vi "ReadData_5782.vi"(10 "Buffer mode":T1, 11 "scope params":T2) -> (0 "error out":errorcluster, 1 "Num elements":i32, 2 "data":dbl[][](array[numeric]) format="%.2f", 3 "scope params out":T2)   [LabVIEW 2013]
uses:
  controls/scope_params_5782.ctl
  Utilities/Ticker/Ticker.lvclass
  Scope/controls/ScopeMode.ctl
  Config/FPGAref_5782.ctl
  FPGA/DataMode.ctl
  controls/5782_trigger_type.ctl
  Scope/controls/Data_display_mode.ctl
  <vilib>/rvi/interface/common/niFpgaWaitOnOcc.vi
  <vilib>/Utility/error.llb/Error Cluster From Error Code.vi
  <vilib>/rvi/errors/niLvFpgaAdjustHostInterfaceError.vi
  <vilib>/rvi/interface/nirviMethod/nirviMethod.xnode
  <vilib>/FPGAPlugInAG/Dynamic/niLvFpga_ReadFifo_Dynamic.vi
  <vilib>/rvi/errors/niLvFpgaMergeErrorWithErrorCode.vi
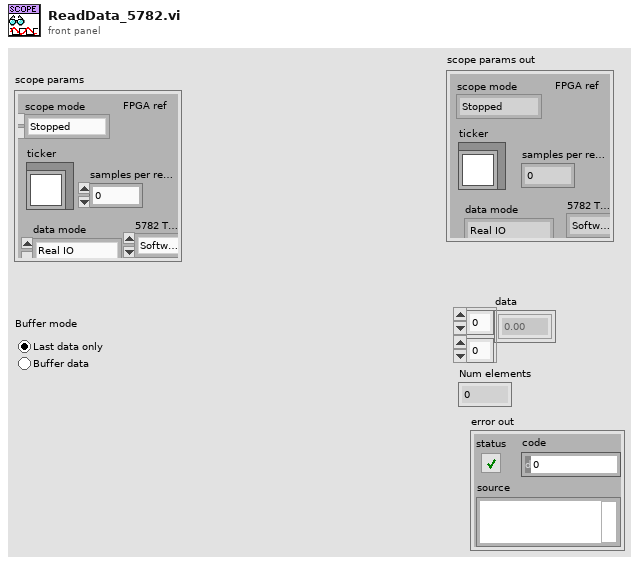
[diagram p1: front panel]
types:
  T1 = typedef "Data_display_mode.ctl" = enum32{"Last data only", "Buffer data"}
  T2 = typedef "scope_params_5782.ctl" = cluster{"scope mode":T3, "ticker":refnum<class "Ticker.lvclass">, "samples per record":i32, "FPGA ref":T4, "data mode":T5, "5782 Trigger":T6, "Chart length":i32}
  T3 = typedef "ScopeMode.ctl" = enum16{"Stopped", "Single", "Running", "Continuous"}
  T4 = typedef "FPGAref_5782.ctl" = refnum<k20>
  T5 = typedef "DataMode.ctl" = enum16{"Real IO", "Simulated"}
  T6 = typedef "5782_trigger_type.ctl" = enum16{"Software", "Trigger input"}
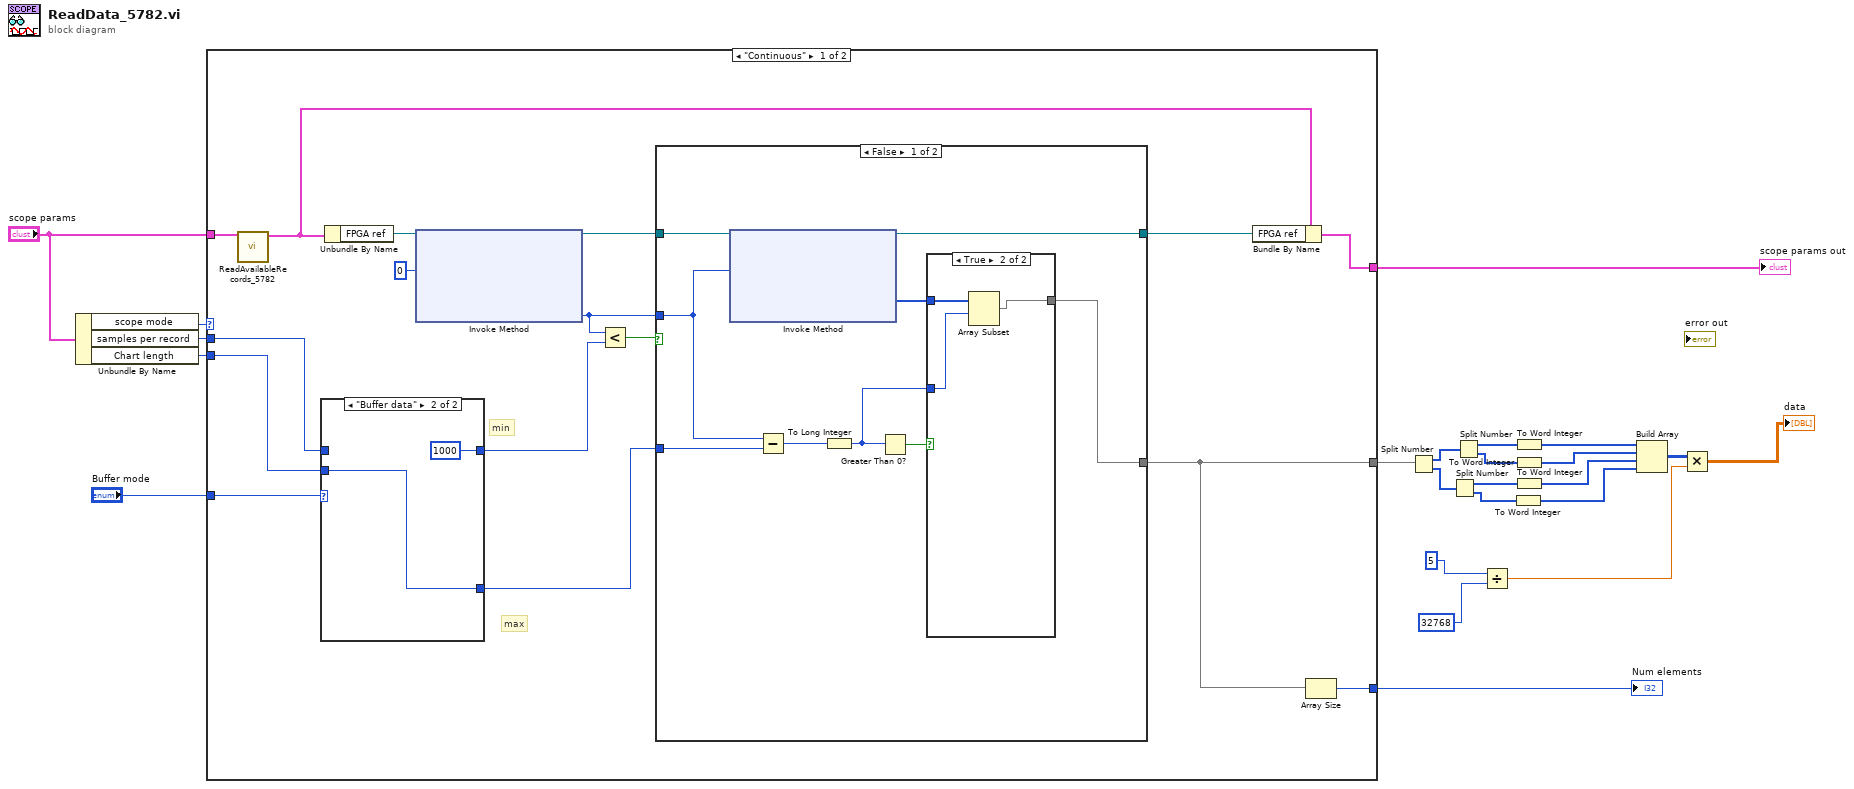
[diagram p0: block diagram]
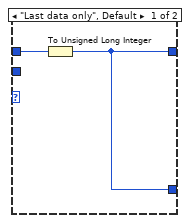
[diagram p4: hidden frame]
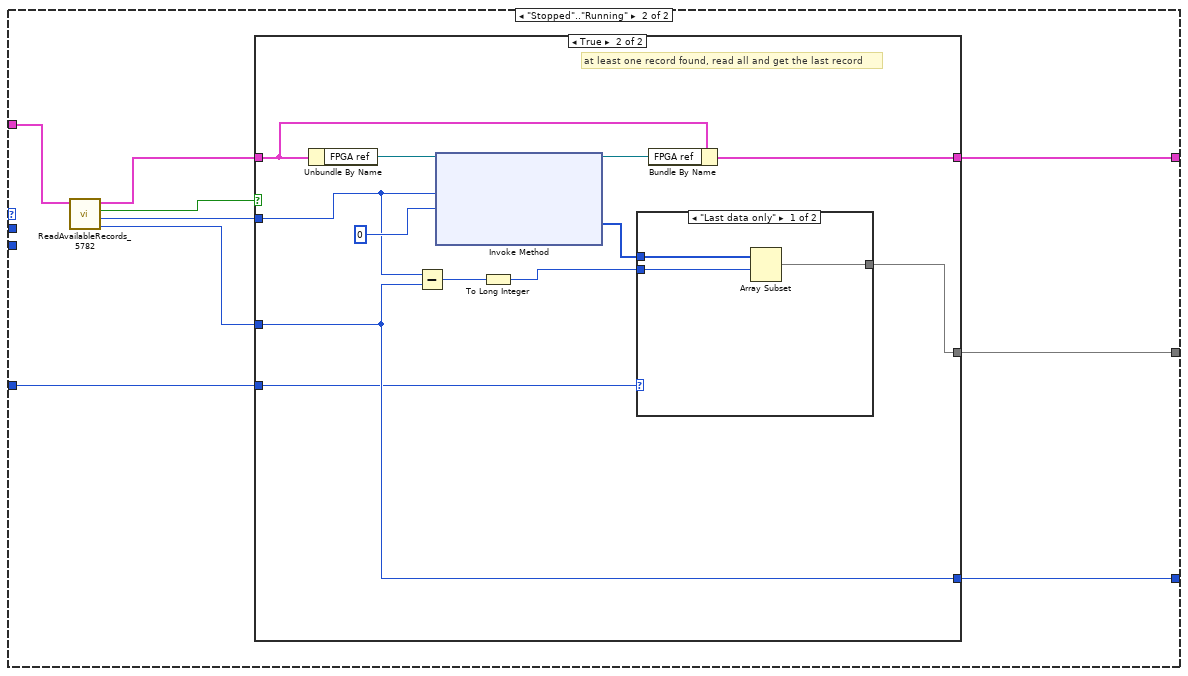
[diagram p5: hidden frame]
diagram:
  n1 = Unbundle By Name("scope params") -> ("scope mode"=w20:T3, "samples per record"=w2:i32, "Chart length"=w1:i32)
  n2 = case shown="\"Continuous\"" w20 {
    tunnel: [w28 w66] -> w23
    tunnel: [w30 w61] -> w22
    tunnel: [w29 w60] -> w4
    tunnel: "scope params" -> [w26 w59]
    tunnel: "Buffer mode" -> [w39 w58]
    tunnel: w2 -> [w27 _]
    tunnel: w1 -> [w24 _]
    frame "Continuous" {
      # "min"
      # "max"
      n3 = call "ReadAvailableRecords_5782.vi"("scope params"=w26) -> ("scope params out"=w25:T2)  [unwired: 7 in, 3 out]
      n4 = case shown="\"Buffer data\"" w39 {
        tunnel: [w54 u32 1000] -> w36
        tunnel: [w54 w56] -> w32
        tunnel: w27 -> [w55 _]
        tunnel: w24 -> [_ w56]
        frame "Last data only", Default {
          n5 = To Unsigned Long Integer(number=w55) -> (unsigned 32bit integer=w54:u32)
        }
        frame "Buffer data" {
        }
      }
      n6 = Unbundle By Name(w25) -> ("FPGA ref"=w38:T4)
      n7 = xnode "Invoke Method"("FPGA VI Reference In"=w38, "Number of Elements"=u32 0) -> ("FPGA VI Reference Out"=w34:T4, "Elements Remaining"=w33:u32)  [unwired: 2 in, 2 out]
      n8 = Less?(x=w33, y=w36) -> (x < y?=w35:bool)
      n9 = case shown="False" w35 {
        tunnel: w34 -> [w48 w53]
        tunnel: w33 -> [w46 _]
        tunnel: w32 -> [w45 _]
        tunnel: [w41 _] -> w29
        tunnel: [w40 w53] -> w31
        frame False {
          n10 = xnode "Invoke Method"("FPGA VI Reference In"=w48, "Number of Elements"=w46) -> ("FPGA VI Reference Out"=w40:T4, "Data"=w43:u64[])  [unwired: 2 in, 2 out]
          n11 = Subtract(x=w46, y=w45) -> (x-y=w47:u32)
          n12 = To Long Integer(number=w47) -> (32bit integer=w42:i32)
          n13 = Greater Than 0?(x=w42) -> (x > 0?=w44:bool)
          n14 = case shown="True" w44 {
            tunnel: w43 -> [w49 w52]
            tunnel: w42 -> [_ w51]
            tunnel: [w49 w50] -> w41
            frame False {
            }
            frame True {
              n15 = Array Subset(array=w52, index=w51) -> (w50:u64[])  [unwired: 1 in]
            }
          }
        }
        frame True {
          # "too few elements"
        }
      }
      n16 = Bundle By Name(cluster=w25, "FPGA ref"=w31) -> (w30:T2)
      n17 = Array Size(array=w29) -> (size(s)=w28:i32)
    }
    frame "Stopped".."Running" {
      n18 = call "ReadAvailableRecords_5782.vi"("scope params"=w59) -> ("last record size"=w63:u32, "#elements"=w64:u32, "record available"=w65:bool, "scope params out"=w62:T2)  [unwired: 7 in]
      n19 = case shown="True" w65 {
        tunnel: [_ w68] -> w60
        tunnel: [_ w71] -> w66
        tunnel: w64 -> [_ w77]
        tunnel: w63 -> [_ w71]
        tunnel: w62 -> [w67 w75]
        tunnel: [w67 w70] -> w61
        tunnel: w58 -> [_ w69]
        frame False {
        }
        frame True {
          # "at least one record found, read all and get the last record"
          n20 = Unbundle By Name(w75) -> ("FPGA ref"=w76:T4)
          n21 = Subtract(x=w77, y=w71) -> (x-y=w73:u32)
          n22 = xnode "Invoke Method"("FPGA VI Reference In"=w76, "Number of Elements"=w77, "Timeout (ms)"=0) -> ("FPGA VI Reference Out"=w74:T4, "Data"=w79:u64[])  [unwired: 1 in, 2 out]
          n23 = To Long Integer(number=w73) -> (32bit integer=w72:i32)
          n24 = case shown="\"Last data only\"" w69 {
            tunnel: w79 -> [w82 w83]
            tunnel: w72 -> [w81 _]
            tunnel: [w80 w83] -> w68
            frame "Last data only" {
              n25 = Array Subset(array=w82, index=w81) -> (w80:u64[])  [unwired: 1 in]
            }
            frame "Buffer data" {
            }
          }
          n26 = Bundle By Name(cluster=w75, "FPGA ref"=w74) -> (w70:T2)
        }
      }
    }
  }
  "scope params out" <- w22
  "Num elements" <- w23
  n27 = Split Number(x=w4) -> (hi(x)=w9:u32[], lo(x)=w5:u32[])
  n28 = Split Number(x=w5) -> (hi(x)=w7:u16[], lo(x)=w8:u16[])
  n29 = Split Number(x=w9) -> (hi(x)=w10:u16[], lo(x)=w6:u16[])
  n30 = Divide(x=5, y=32768) -> (x/y=w18:dbl)
  n31 = To Word Integer(number=w8) -> (16bit integer=w14:i16[])
  n32 = To Word Integer(number=w10) -> (16bit integer=w11:i16[])
  n33 = To Word Integer(number=w6) -> (16bit integer=w12:i16[])
  n34 = To Word Integer(number=w7) -> (16bit integer=w13:i16[])
  n35 = Build Array(w11, w12, w13, w14) -> (w15:i16[][])
  n36 = Multiply(x=w15, y=w18) -> (x*y=→"data":dbl[][])
